vi "Get dcvmDPI_InitializeRequest.vi"(8 "error in (no error)":errorcluster, 11 "gRPCid":T2) -> (0 "error out":errorcluster, 2 "package_templatemessage":T1, 3 "gRPCid out":T2)   [LabVIEW 2021, in "dcvmDPI_AD7606B_server.lvlib"]
uses:
  dcvmDPI_AD7606B_server.lvlib
  <vilib>/gRPC/LabVIEW gRPC Library/Shared/grpcId.ctl
  dcvmDPI_InitializeRequest.ctl
  a51dd2a7-b5c1-4c09-9df4-8cd9d3bd0c19.vi
  <vilib>/gRPC/LabVIEW gRPC Library/Shared/TranslateGrpcError.vi
  <vilib>/gRPC/LabVIEW gRPC Library/Server API/Server/Get Server DLL Path.vi
  <vilib>/Utility/error.llb/Error Cluster From Error Code.vi
  <vilib>/gRPC/LabVIEW gRPC Library/grpc-lvsupport-release.lvlib
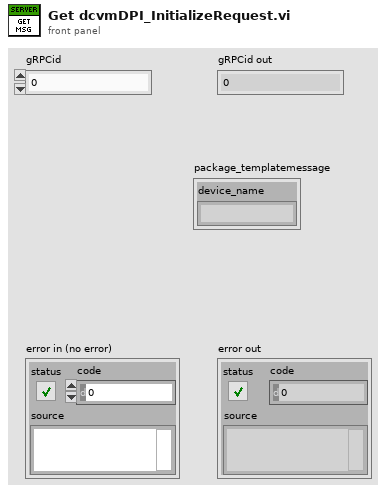
[diagram p1: front panel]
types:
  T1 = typedef "dcvmDPI_AD7606B_server.lvlib/dcvmDPI_InitializeRequest.ctl" = cluster{"device_name":string}
  T2 = typedef "grpc-lvsupport-release.lvlib/grpcId.ctl" = u64
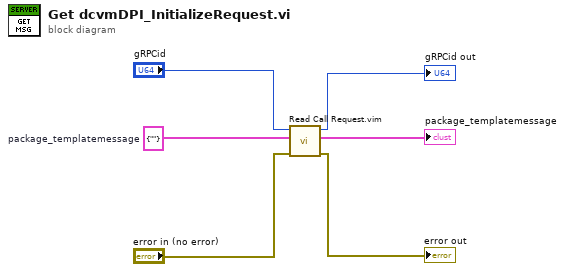
[diagram p0: block diagram]
diagram:
  w2 = T1 {"device_name"=""}  # package_templatemessage
  n1 = call "Read Call Request.vim"("error in"="error in (no error)", "Request Type"=w2, "gRPCid in"="gRPCid") -> ("error out"=→"error out":errorcluster, "Request Data"=→"package_templatemessage":T1, "gRPCid out"=→"gRPCid out":T2)  [unwired: 6 in]
